vi "ADCP_Processed_Bytes_To_CM_Packet.vi"(8 "error in (no error)":errorcluster, 10 "Processed Packet Bytes":u8[](array[numeric]), 11 "ADCP In":refnum<class "ADCP.lvclass">) -> (0 "error out":errorcluster, 2 "CM Packet":T1, 3 "ADCP out":refnum<class "ADCP.lvclass">)   [LabVIEW 2017, in "ADCP.lvclass"]
uses:
  ADCP.lvclass
  ADCP.lvclass/ADCP.ctl
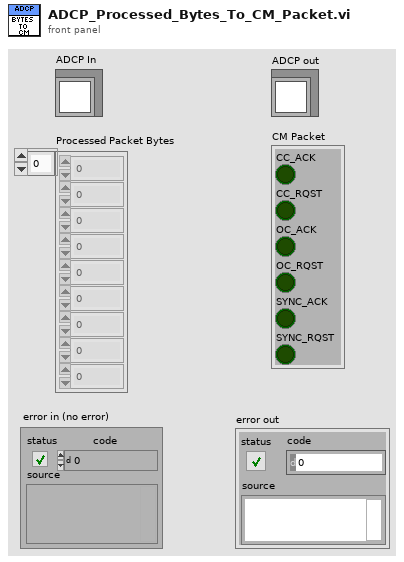
[diagram p1: front panel]
types:
  T1 = cluster{"CC_ACK":bool, "CC_RQST":bool, "OC_ACK":bool, "OC_RQST":bool, "SYNC_ACK":bool, "SYNC_RQST":bool}
  T2 = enum16{"Data", "Connection Management", "Remote Request", "Error and status", "INVALID"}
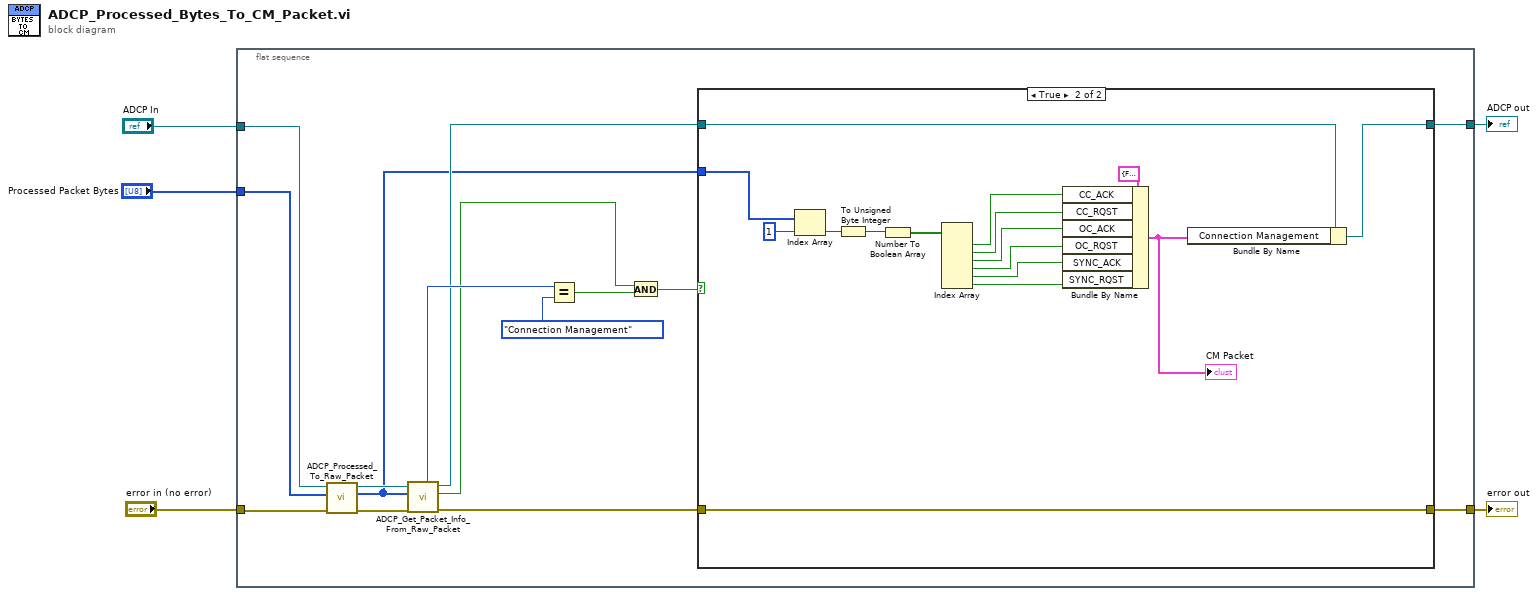
[diagram p0: block diagram]
diagram:
  n1 = flat-sequence {
    tunnel: "ADCP In" -> [w19]
    tunnel: "error in (no error)" -> [w20]
    tunnel: "Processed Packet Bytes" -> [w18]
    tunnel: [w8] -> w2
    tunnel: [w7] -> w1
    frame #0 {
      n2 = call "ADCP_Processed_To_Raw_Packet.vi"("error in (no error)"=w20, "Processed Packet"=w18, "ADCP in"=w19) -> ("error out"=w16:errorcluster, "Raw Packet"=w6:u8[], "ADCP out"=w17:refnum<class "ADCP.lvclass">)  [unwired: 6 in]
      n3 = call "ADCP_Get_Packet_Info_From_Raw_Packet.vi"("error in (no error)"=w16, "Raw Packet"=w6, "ADCP in"=w17) -> ("error out"=w11:errorcluster, "Checksum Valid ?"=w12:bool, "ADCP out"=w9:refnum<class "ADCP.lvclass">, "Packet Type"=w15:T2)  [unwired: 2 in, 3 out]
      n4 = Equal?(x=w15, y=T2."Connection Management") -> (x = y?=w13:bool)
      n5 = And(x=w12, y=w13) -> (x .and. y?=w10:bool)
      n6 = case shown="True" w10 {
        tunnel: w11 -> [w21 w23]
        tunnel: w9 -> [w22 w33]
        tunnel: [w22 w32] -> w8
        tunnel: [w21 w23] -> w7
        tunnel: w6 -> [_ w38]
        frame False {
        }
        frame True {
          n7 = Index Array(array=w38, index=1) -> (element=w36:u8)
          n8 = To Unsigned Byte Integer(number=w36) -> (unsigned 8bit integer=w35:u8)
          n9 = Number To Boolean Array(number=w35) -> (Boolean array=w34:bool[])
          n10 = Index Array(array=w34) -> (element #1=w30:bool, element #2=w28:bool, element #3=w27:bool, element #4=w26:bool, element #5=w25:bool, element #6=w24:bool)  [unwired: 6 in]
          n11 = Bundle By Name(cluster=T1 {"CC_ACK"=FALSE, "CC_RQST"=FALSE, "OC_ACK"=FALSE, "OC_RQST"=FALSE, "SYNC_ACK"=FALSE, "SYNC_RQST"=FALSE} ("Connection Management"), "CC_ACK"=w30, "CC_RQST"=w28, "OC_ACK"=w27, "OC_RQST"=w26, "SYNC_ACK"=w25, "SYNC_RQST"=w24) -> (w29:T1)
          "CM Packet" <- w29
          n12 = Bundle By Name(cluster=w33, "Connection Management"=w29) -> (w32:refnum<class "ADCP.lvclass">)
        }
      }
    }
  }
  "ADCP out" <- w2
  "error out" <- w1
